vi "child.vi"   [LabVIEW 2009]
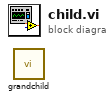
[diagram p0: block diagram]
diagram:
  n1 = call "grandchild.vi"() -> ()  [unwired: 1 in]
